vi "CRYGet Curve Library Data.vi"(0 "Type":enum16{"Curves", "Values", "Results", "WFM"}(ring), 1 "Data Name":string) -> (2 "Step No.":i32, 3 "Curve":T2={"Name"="", "Curve"=[], "X data"=1, "Y data"=1, "Z data"=1, "X axis"=0, "Y axis"=1, "Z axis"=1, "X unit"="Hz", "Y unit"="", "Z unit"="deg.", "X dB ref"=1.0, "Y dB ref"=1.0, "Z dB ref"=1.0, "single val"=FALSE, "protected"=FALSE, "display X"=TRUE, "display Y"=TRUE, "display Z"=TRUE, "Test Info"="", "Step No."=0, "Plot Settings"={"Color"=0, "Interpolation"=0, "Point Style"=0, "Line Style"=0, "Point Color"=0, "Line Width"=0, "Bar Plot Style"=0, "Fill To"=0}, "AutoProtect"=FALSE} {"Z data" items=["dB", "Lin"]; "X data" items=["dB", "Lin"]; "Y data" items=["dB", "Lin"]; "Z dB ref" format="%.1f"; "Z axis" items=["Log", "Lin"]; "X dB ref" format="%.1f"; "X axis" items=["Log", "Lin"]; "Y axis" items=["Log", "Lin"]; "Y dB ref" format="%.1f"; "Curve"."z" format="%.2f"; "Curve"."y" format="%.2f"; "Curve"."x" format="%.2f"}, 4 "Value":T2={"Name"="", "Curve"=[], "X data"=1, "Y data"=1, "Z data"=1, "X axis"=0, "Y axis"=1, "Z axis"=1, "X unit"="Hz", "Y unit"="", "Z unit"="deg.", "X dB ref"=1.0, "Y dB ref"=1.0, "Z dB ref"=1.0, "single val"=FALSE, "protected"=FALSE, "display X"=TRUE, "display Y"=TRUE, "display Z"=TRUE, "Test Info"="", "Step No."=0, "Plot Settings"={"Color"=0, "Interpolation"=0, "Point Style"=0, "Line Style"=0, "Point Color"=0, "Line Width"=0, "Bar Plot Style"=0, "Fill To"=0}, "AutoProtect"=FALSE} {"Z data" items=["dB", "Lin"]; "X data" items=["dB", "Lin"]; "Y data" items=["dB", "Lin"]; "Z dB ref" format="%.1f"; "Z axis" items=["Log", "Lin"]; "X dB ref" format="%.1f"; "X axis" items=["Log", "Lin"]; "Y axis" items=["Log", "Lin"]; "Y dB ref" format="%.1f"; "Curve"."z" format="%.2f"; "Curve"."y" format="%.2f"; "Curve"."x" format="%.2f"}, 5 "Wave":T3={"Waveform"={"X0"=0.0, "dX"=0.0, "Y"=[]}, "X data"=1, "Y data"=0, "Y axis"=0, "X unit"="s", "Y unit"="", "Y dB ref"=1.0, "display Y"=TRUE, "display X"=FALSE, "Overload?"=FALSE, "Test Info"="", "Step No."=0, "Name"="", "protected"=FALSE, "Sqc history"=[], "Signal Channel ID"=0, "Plot Settings"={"Color"=0, "Interpolation"=0, "Point Style"=0, "Line Style"=0, "Point Color"=0, "Line Width"=0, "Bar Plot Style"=0, "Fill To"=0}, "AutoProtect"=FALSE} {"Y dB ref" format="%.1f"; "Y axis" items=["Log", "Lin"]; "Y data" items=["dB", "Lin"]; "X data" items=["dB", "Lin"]}, 6 "index":i32)   [LabVIEW 2013]
uses:
  CRYSystem/Typedef Control/CRYWaveform Cluster.ctl
  CRYSystem/Typedef Control/CRYData Cluster.ctl
  CRYSystem/Typedef Control/CRYResult Cluster.ctl
  CRYProject/CRYProject Editor Global.vi
panel:
  out "Result":T1={"Name"="Test for Signal [L]", "Margin"=nan, "unit"="", "Verdict"=FALSE, "Limit"="", "Max/Min"="", "protected"=FALSE, "Step No."=0, "Test Info"="", "AutoProtect"=FALSE} {"Margin" format="%.2f"}
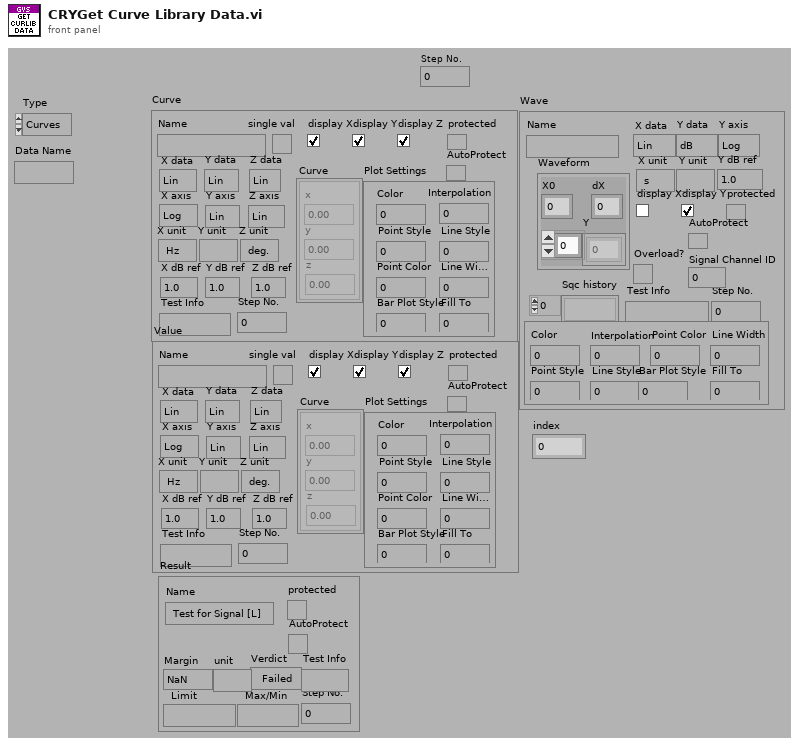
[diagram p1: front panel]
types:
  T1 = typedef "CRYResult Cluster.ctl" = cluster{"Name":string, "Margin":dbl, "unit":string, "Verdict":bool, "Limit":string, "Max/Min":string, "protected":bool, "Step No.":i32, "Test Info":string, "AutoProtect":bool}
  T2 = typedef "CRYData Cluster.ctl" = cluster{"Name":string, "Curve":cluster{"x":dbl, "y":dbl, "z":dbl}[], "X data":u16, "Y data":u16, "Z data":u16, "X axis":u16, "Y axis":u16, "Z axis":u16, "X unit":string, "Y unit":string, "Z unit":string, "X dB ref":dbl, "Y dB ref":dbl, "Z dB ref":dbl, "single val":bool, "protected":bool, "display X":bool, "display Y":bool, "display Z":bool, "Test Info":string, "Step No.":i32, "Plot Settings":cluster{"Color":u32, "Interpolation":u8, "Point Style":u8, "Line Style":u8, "Point Color":u32, "Line Width":u8, "Bar Plot Style":u8, "Fill To":i16}, "AutoProtect":bool}
  T3 = typedef "CRYWaveform Cluster.ctl" = cluster{"Waveform":cluster{"X0":dbl, "dX":dbl, "Y":sgl[]}, "X data":u16, "Y data":u16, "Y axis":u16, "X unit":string, "Y unit":string, "Y dB ref":dbl, "display Y":bool, "display X":bool, "Overload?":bool, "Test Info":string, "Step No.":i32, "Name":string, "protected":bool, "Sqc history":string[], "Signal Channel ID":i32, "Plot Settings":cluster{"Color":u32, "Interpolation":u8, "Point Style":u8, "Line Style":u8, "Point Color":u32, "Line Width":u8, "Bar Plot Style":u8, "Fill To":i16}, "AutoProtect":bool}
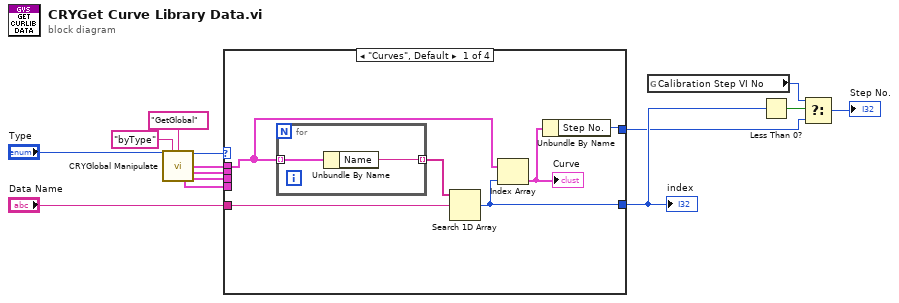
[diagram p0: block diagram]
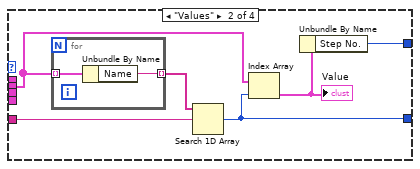
[diagram p2: hidden frame]
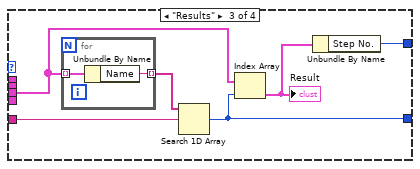
[diagram p3: hidden frame]
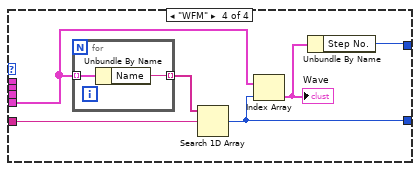
[diagram p4: hidden frame]
diagram:
  n1 = call "CRYGlobal Manipulate.vi"("Type"="Type", "sOption"="byType", "sAction"="GetGlobal") -> ("Type out"=w13:enum16{"Curves", "Values", "Results", "WFM"}, "Curves Out"=w11:T2[], "Values Out"=w10:T2[], "WFM Out"=w8:T3[], "Results Out"=w9:T1[])  [unwired: 6 in, 2 out]
  n2 = case shown="\"Curves\", Default" w13 {
    tunnel: "Data Name" -> [w20 w28 w34 w43]
    tunnel: [w18 w27 w35 w42] -> w5
    tunnel: [w16 w24 w32 w40] -> w3
    tunnel: w11 -> [w15 _ _ _]
    tunnel: w10 -> [_ w23 _ _]
    tunnel: w9 -> [_ _ w31 _]
    tunnel: w8 -> [_ _ _ w39]
    frame "Curves", Default {
      n3 = for {
        tunnel: w15 -> [w22] mode=indexing
        tunnel: [w21] -> w19 mode=indexing
        n4 = Unbundle By Name(w22) -> ("Name"=w21:string)
      }
      n5 = Search 1D Array(1D array=w19, element=w20) -> (index of element=w18:i32)  [unwired: 1 in]
      n6 = Index Array(array=w15, index=w18) -> (element=w17:T2)
      "Curve" <- w17
      n7 = Unbundle By Name(w17) -> ("Step No."=w16:i32)
    }
    frame "Values" {
      n8 = for {
        tunnel: w23 -> [w30] mode=indexing
        tunnel: [w29] -> w26 mode=indexing
        n9 = Unbundle By Name(w30) -> ("Name"=w29:string)
      }
      n10 = Search 1D Array(1D array=w26, element=w28) -> (index of element=w27:i32)  [unwired: 1 in]
      n11 = Index Array(array=w23, index=w27) -> (element=w25:T2)
      "Value" <- w25
      n12 = Unbundle By Name(w25) -> ("Step No."=w24:i32)
    }
    frame "Results" {
      n13 = for {
        tunnel: w31 -> [w38] mode=indexing
        tunnel: [w37] -> w36 mode=indexing
        n14 = Unbundle By Name(w38) -> ("Name"=w37:string)
      }
      n15 = Search 1D Array(1D array=w36, element=w34) -> (index of element=w35:i32)  [unwired: 1 in]
      n16 = Index Array(array=w31, index=w35) -> (element=w33:T1)
      "Result" <- w33
      n17 = Unbundle By Name(w33) -> ("Step No."=w32:i32)
    }
    frame "WFM" {
      n18 = for {
        tunnel: w39 -> [w46] mode=indexing
        tunnel: [w45] -> w44 mode=indexing
        n19 = Unbundle By Name(w46) -> ("Name"=w45:string)
      }
      n20 = Search 1D Array(1D array=w44, element=w43) -> (index of element=w42:i32)  [unwired: 1 in]
      n21 = Index Array(array=w39, index=w42) -> (element=w41:T3)
      "Wave" <- w41
      n22 = Unbundle By Name(w41) -> ("Step No."=w40:i32)
    }
  }
  "index" <- w5
  n23 = global read "CRYProject Editor Global.vi" "Calibration Step VI No"() -> (w2:i32)
  n24 = Less Than 0?(x=w5) -> (x < 0?=w4:bool)
  n25 = Select(t=w2, s=w4, f=w3) -> (s? t:f=→"Step No.":i32)
